vi "PPSsync.vi"(5 "Halt":bool, 6 "Advance":bool) -> (1 "PPS":bool, 2 "Timekeeper Locked":bool)   [LabVIEW 2015]
uses:
  PPS_Global_Var.vi
  Supporting Files/test_sup.vi
  <vilib>/Utility/error.llb/Error Cluster From Error Code.vi
  <vilib>/rvi/errors/niLvFpgaAdjustHostInterfaceError.vi
  <vilib>/rvi/interface/nirviReadWriteControl/nirviReadWriteControl.xnode
  NiFpgaLv.dll
  <vilib>/rvi/interface/Simulation/niFpgaSimulationCallBeginRW.vi
panel:
  out "Epoch Time (ref)":dbl
  out "Offset (ns)":dbl
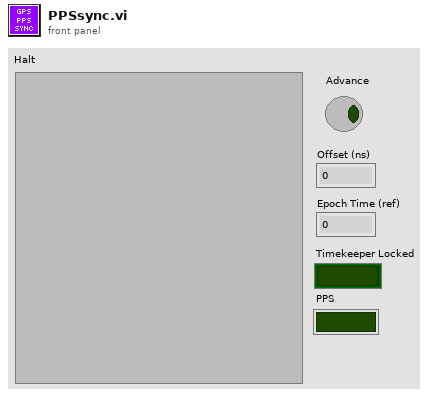
[diagram p1: front panel]
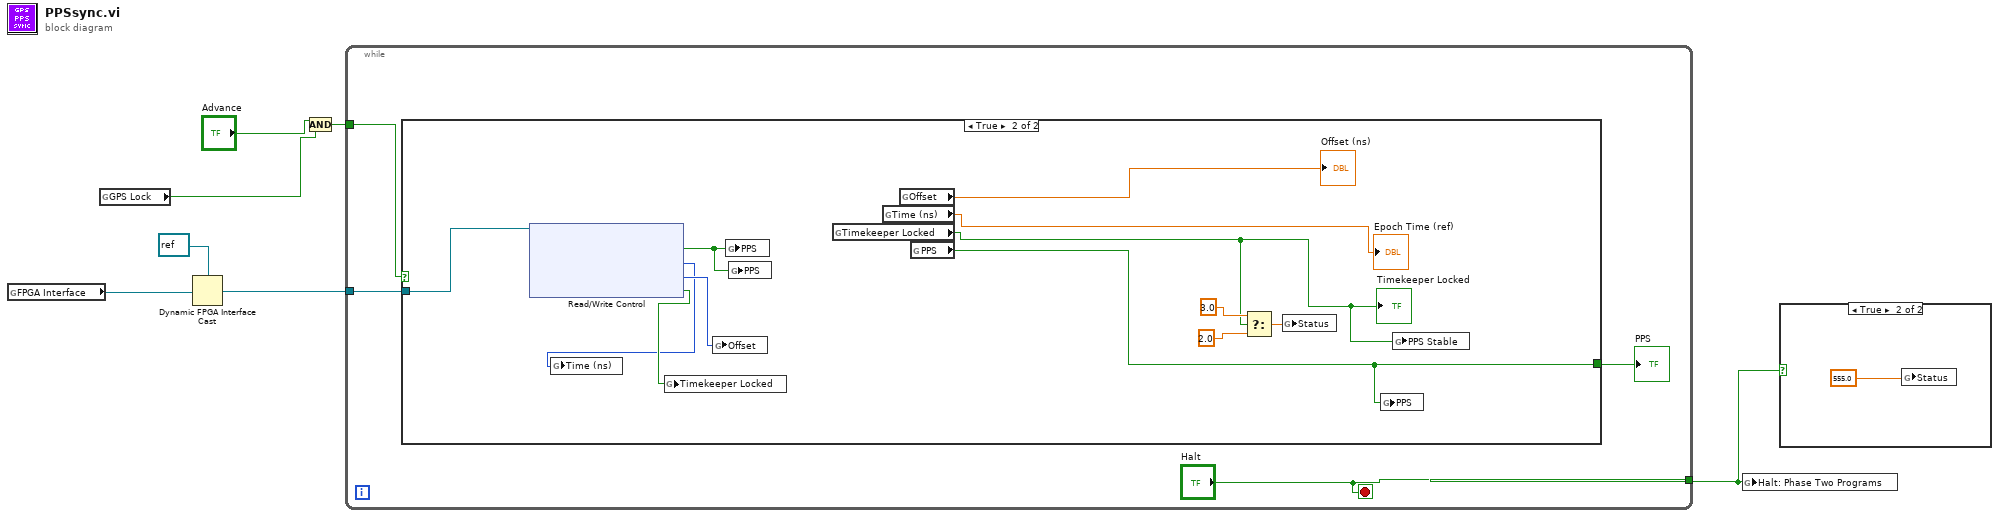
[diagram p0: block diagram]
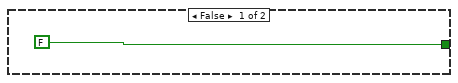
[diagram p3: hidden frame]
diagram:
  n1 = global read "test_sup.vi" "FPGA Interface"() -> (w2:refnum<k20>)
  n2 = global read "PPS_Global_Var.vi" "GPS Lock"() -> (w3:bool)
  n3 = Dynamic FPGA Interface Cast(Session In=refnum<k20> refnum ("FPGA Interface"), Type=w2) -> (Session Out=w4:refnum<k20>)
  n4 = And(x="Advance", y=w3) -> (x .and. y?=w7:bool)
  n5 = while {
    tunnel: w7 -> [w11]
    tunnel: ["Halt"] -> w1
    tunnel: w4 -> [w8]
    stop <- "Halt" stop-if-true
    n6 = case shown="True" w11 {
      tunnel: [FALSE w18] -> w9
      tunnel: w8 -> [_ w13]
      frame False {
      }
      frame True {
        n7 = xnode "Read/Write Control"("FPGA VI Reference In"=w13) -> ("PPS"=w14:bool, "FPGA Timekeeper time (ns)"=w15:u64, "offset from time reference"=w17:i32, "FPGA Timekeeper locked"=w16:bool)  [unwired: 1 in, 2 out]
        n8 = global write "test_sup.vi" "Time (ns)"(w15) -> ()
        n9 = global write "test_sup.vi" "Timekeeper Locked"(w16) -> ()
        n10 = global write "test_sup.vi" "Offset"(w17) -> ()
        n11 = global write "PPS_Global_Var.vi" "PPS"(w14) -> ()
        n12 = global write "test_sup.vi" "PPS"(w14) -> ()
        n13 = global read "test_sup.vi" "Timekeeper Locked"() -> (w19:bool)
        "Timekeeper Locked" <- w19
        n14 = global read "test_sup.vi" "Time (ns)"() -> (→"Epoch Time (ref)":dbl)
        n15 = global read "test_sup.vi" "Offset"() -> (→"Offset (ns)":dbl)
        n16 = global read "test_sup.vi" "PPS"() -> (w18:bool)
        n17 = Select(t=3.0, s=w19, f=2.0) -> (s? t:f=w24:dbl)
        n18 = global write "PPS_Global_Var.vi" "Status"(w24) -> ()
        n19 = global write "PPS_Global_Var.vi" "PPS"(w18) -> ()
        n20 = global write "PPS_Global_Var.vi" "PPS Stable"(w19) -> ()
      }
    }
    "PPS" <- w9
  }
  n21 = global write "PPS_Global_Var.vi" "Halt: Phase Two Programs"(w1) -> ()
  n22 = case shown="True" w1 {
    frame False {
    }
    frame True {
      n23 = global write "PPS_Global_Var.vi" "Status"(555.0) -> ()
    }
  }
